vi "Speed Adjustment.vi"(0 "spectrum information":T3={"spectrum"={"f0"=0.0, "df"=0.1, "magnitude [dB]"=[]}, "demodulated? (F)"=FALSE}, 1 "fundamental frequency [Hz]":dbl, 7 "max sideband order (1)":u8=1, 11 "error in (no error)":errorcluster, 12 "candidate speeds":cluster{"speed [RPM]":dbl, "slip":dbl}[](array[cluster]), 13 "nameplate information":T1) -> (3 "slip":dbl, 4 "upper sidebands":T2, 6 "lower sidebands":T2, 8 "max sideband magnitude [dB]":dbl, 10 "speed [RPM]":dbl, 15 "error out":errorcluster)   [LabVIEW 2017]
uses:
  <vilib>/addons/Electrical Power/Motor Monitoring/Broken Rotor Bar Harmonics (1 Motor).vi
  <vilib>/addons/Electrical Power/Motor Monitoring/NI_EP_Motor Monitoring.lvlib
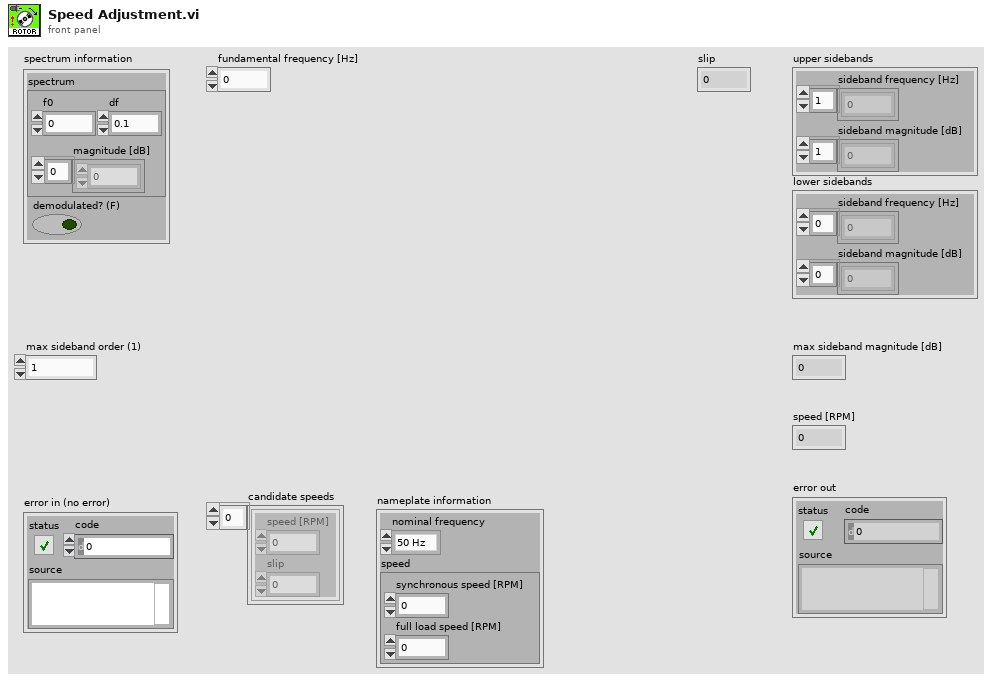
[diagram p1: front panel]
types:
  T1 = cluster{"nominal frequency":enum16{"50 Hz", "60 Hz"}, "speed":cluster{"synchronous speed [RPM]":dbl, "full load speed [RPM]":dbl}}
  T2 = cluster{"sideband frequency [Hz]":dbl[], "sideband magnitude [dB]":dbl[]}
  T3 = cluster{"spectrum":cluster{"f0":dbl, "df":dbl, "magnitude [dB]":dbl[]}, "demodulated? (F)":bool}
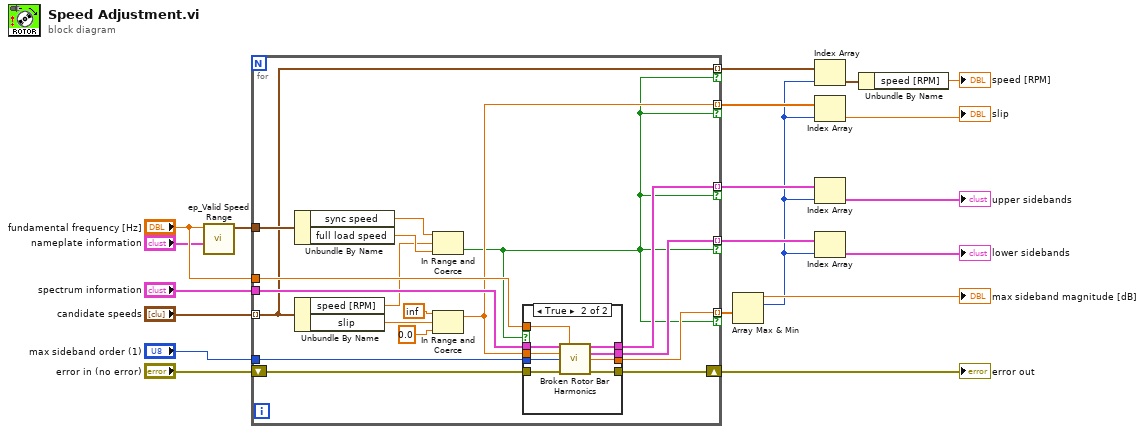
[diagram p0: block diagram]
diagram:
  n1 = call "ep_Valid Speed Range.vi"("nameplate information"="nameplate information", "fundamental frequency [Hz]"="fundamental frequency [Hz]") -> ("speed range [RPM]"=w6:cluster{"sync speed":dbl, "full load speed":dbl})  [unwired: 8 in, 1 out]
  n2 = for {
    tunnel: "candidate speeds" -> [w23] mode=indexing
    tunnel: "spectrum information" -> [w38]
    tunnel: "fundamental frequency [Hz]" -> [w37]
    shift-right: [w35] -> w16
    shift-left: "error in (no error)" -> [w36]
    tunnel: w6 -> [w31]
    tunnel: [w27] -> w15 mode=indexing if=w21
    tunnel: [w26] -> w12 mode=indexing if=w21
    tunnel: [w25] -> w9 mode=indexing if=w21
    tunnel: [w23] -> w13 mode=indexing if=w21
    tunnel: "max sideband order (1)" -> [w24]
    tunnel: [w22] -> w3 mode=indexing if=w21
    n3 = Unbundle By Name(w31) -> ("sync speed"=w30:dbl, "full load speed"=w29:dbl)
    n4 = Unbundle By Name(w23) -> ("speed [RPM]"=w28:dbl, "slip"=w34:dbl)
    n5 = In Range and Coerce(upper limit=w30, x=w28, lower limit=w29) -> (In Range?=w21:bool)  [unwired: 1 out]
    n6 = In Range and Coerce(upper limit=inf, x=w34, lower limit=0.0) -> (coerced(x)=w22:dbl)  [unwired: 1 out]
    n7 = case shown="True" w21 {
      tunnel: w38 -> [_ w48]
      tunnel: w37 -> [_ w47]
      tunnel: w36 -> [w39 w46]
      tunnel: [w39 w45] -> w35
      tunnel: [_ w44] -> w27
      tunnel: [_ w43] -> w26
      tunnel: [_ w42] -> w25
      tunnel: w24 -> [_ w41]
      tunnel: w22 -> [_ w40]
      frame False {
      }
      frame True {
        n8 = call-poly <vilib>:"Broken Rotor Bar Harmonics.vi"("spectrum information"=w48, "fundamental frequency [Hz]"=w47, "slip"=w40, "max sideband order (10)"=w41, "error in (no error)"=w46) -> ("upper sidebands"=w43:T2, "lower sidebands"=w42:T2, "max sideband magnitude [dB]"=w44:dbl, "error out"=w45:errorcluster)  [unwired: 7 in]
      }
    }
  }
  "error out" <- w16
  n9 = Array Max & Min(array=w15) -> (max value=→"max sideband magnitude [dB]":dbl, max index (indices)=w2:i32)  [unwired: 2 out]
  n10 = Index Array(array=w13, index=w2) -> (element=w19:cluster{"speed [RPM]":dbl, "slip":dbl})
  n11 = Index Array(array=w3, index=w2) -> (element=→"slip":dbl)
  n12 = Index Array(array=w12, index=w2) -> (element=→"upper sidebands":T2)
  n13 = Index Array(array=w9, index=w2) -> (element=→"lower sidebands":T2)
  n14 = Unbundle By Name(w19) -> ("speed [RPM]"=→"speed [RPM]":dbl)
